vi "shift currents.vi"(7 "Combo Box":string(combo), 10 "current in":dbl) -> (2 "current out":dbl)   [LabVIEW 2016, in "sub-VIs.lvlib"]
uses:
  sub-VIs/sub-VIs.lvlib
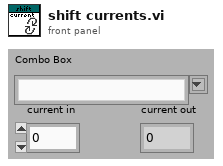
[diagram p1: front panel]
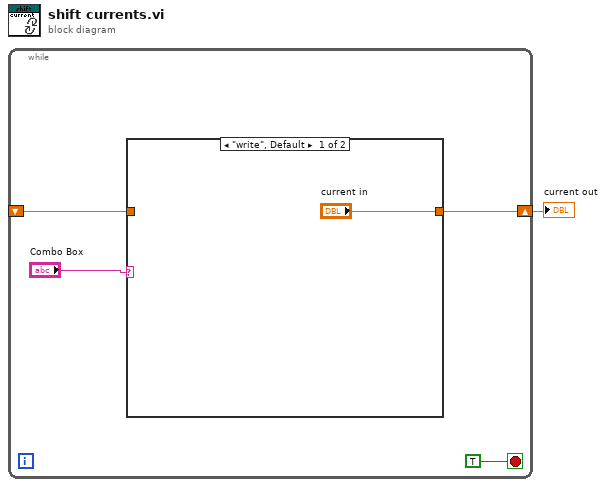
[diagram p0: block diagram]
diagram:
  n1 = while {
    shift-right: [w4] -> w1
    shift-left: _ -> [w3]
    stop <- TRUE stop-if-true
    n2 = case shown="\"write\", Default" "Combo Box" {
      tunnel: ["current in" w7] -> w4
      tunnel: w3 -> [_ w7]
      frame "write", Default {
      }
      frame "read" {
      }
    }
  }
  "current out" <- w1
